vi "Log Data.vi"(8 "error in (no error)":errorcluster, 10 "Message":string, 11 "UserInterface in":refnum<class "UserInterface.lvclass">) -> (0 "error out":errorcluster, 3 "UserInterface out":refnum<class "UserInterface.lvclass">)   [LabVIEW 2022 SP3, in "UserInterface.lvlib" / "UserInterface.lvclass"]
uses:
  UserInterface.lvclass
  UserInterface.lvclass/UserInterface.ctl
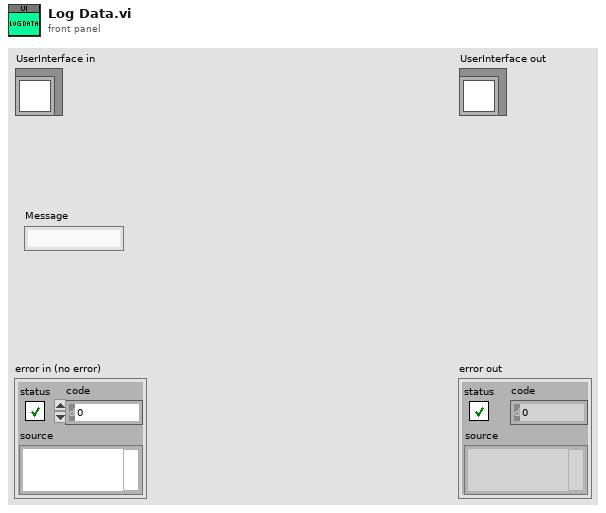
[diagram p1: front panel]
types:
  T1 = cluster{"Image List":refnum<vi>, "ProgressBar":refnum<vi>, "Log":refnum<vi>, "Image Indicator":refnum<vi>}
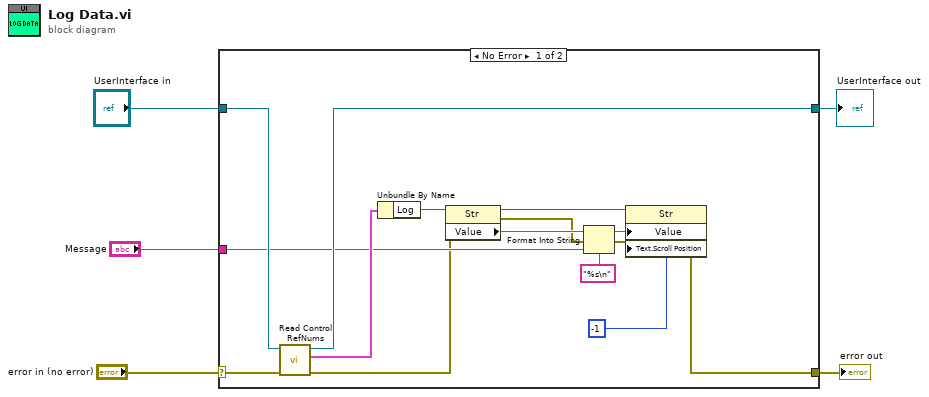
[diagram p0: block diagram]
diagram:
  n1 = case shown="No Error" "error in (no error)" {
    selector: "error in (no error)" -> [w18 w22]
    tunnel: [w7 w22] -> w4
    tunnel: [w19 w21] -> w2
    tunnel: "UserInterface in" -> [w20 w21]
    tunnel: "Message" -> [w12 _]
    frame No Error {
      n2 = call "Read Control RefNums.vi"("error in (no error)"=w18, "UserInterface in"=w20) -> ("error out"=w8:errorcluster, "Control RefNums"=w17:T1, "UserInterface out"=w19:refnum<class "UserInterface.lvclass">)  [unwired: 7 in]
      n3 = Unbundle By Name(w17) -> ("Log"=w16:refnum<vi>)
      n4 = property class="Str"(reference=w16, error in=w8) -> (reference out=w10:refnum<vi>, error out=w13:errorcluster, "Value"=w15:string)
      n5 = Format Into String(format string="%s\n", initial string=w15, error in=w13, w12) -> (resulting string=w9:string, error out=w11:errorcluster)
      n6 = property class="Str"(reference=w10, error in=w11, "Value"=w9, "Text.Scroll Position"=-1) -> (error out=w7:errorcluster)  [unwired: 1 out]
    }
    frame Error {
    }
  }
  "error out" <- w4
  "UserInterface out" <- w2
